vi "Check VISA instrument.vi"(8 "error in (no error)":errorcluster, 10 "visa instrumnet string":string) -> (0 "error out":errorcluster, 3 "error":bool caption="error indicator")   [LabVIEW 2021]
uses:
  <vilib>/regexp/Match Regular Expression.xnode
panel:
  out "device response":string
  out "Read ∆ Time (ms)":dbl format="%.4f"
  out "identifier string":string
  out "VISA instruments":refnum<visa-resource-name>
  in  "included VISA instruments":string[](array[string])=["gpib", "asrl", "com", "end of list"]
  # "end of list should be the last item"
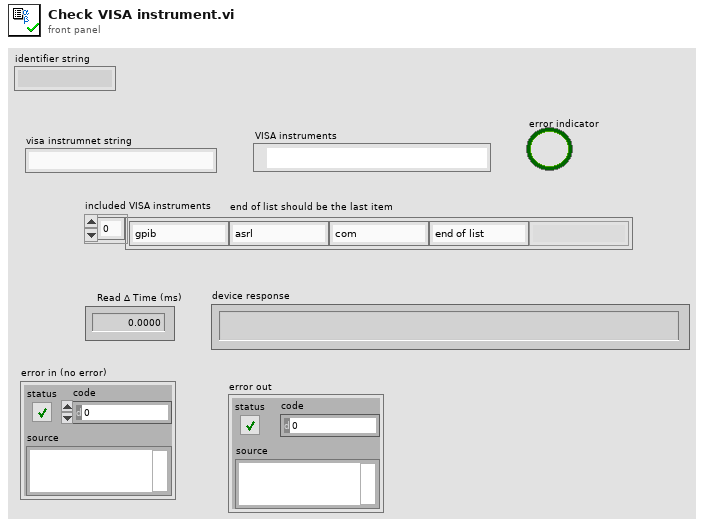
[diagram p1: front panel]
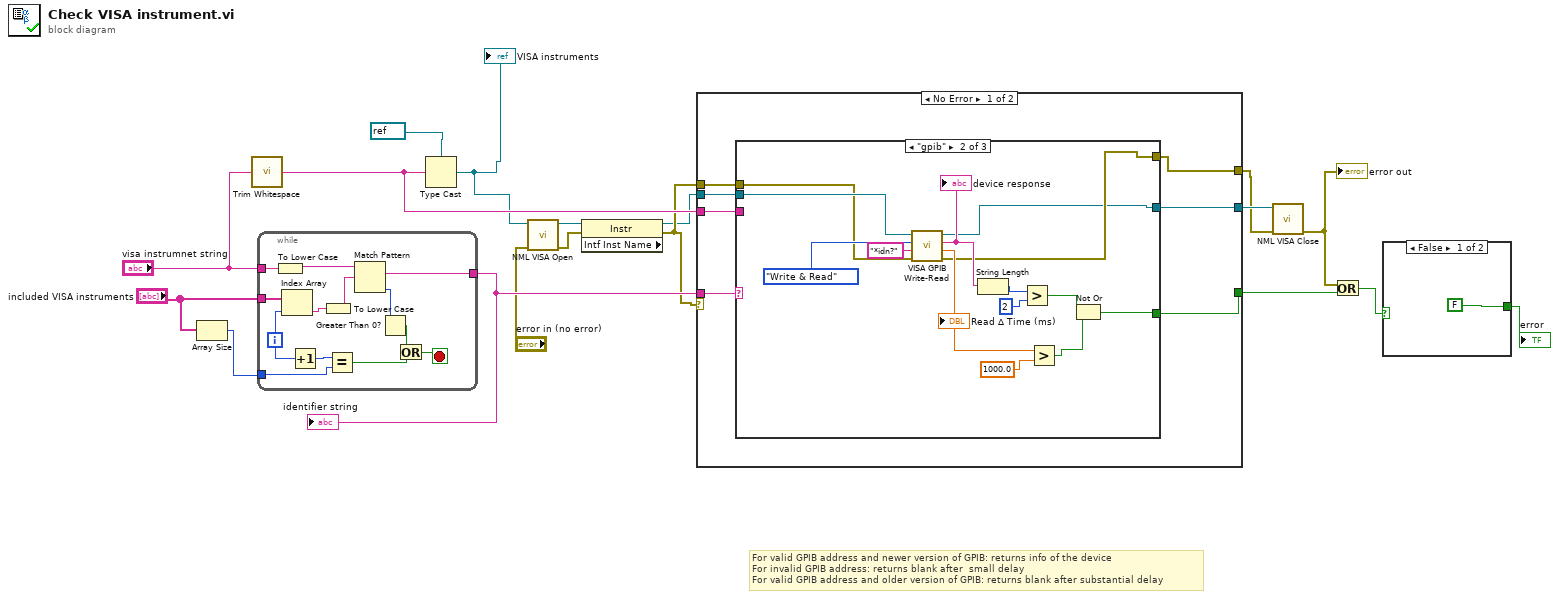
[diagram p0: block diagram]
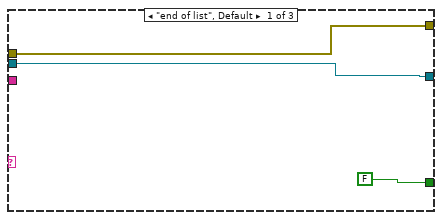
[diagram p2: hidden frame]
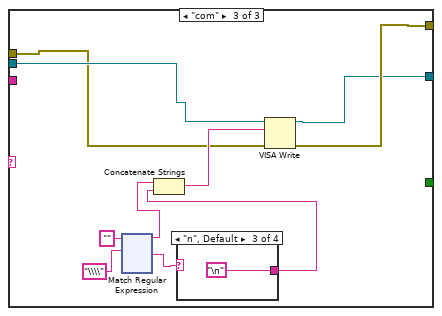
[diagram p3: hidden frame]
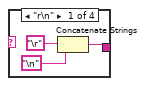
[diagram p4: hidden frame]
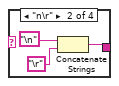
[diagram p5: hidden frame]
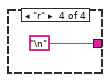
[diagram p6: hidden frame]
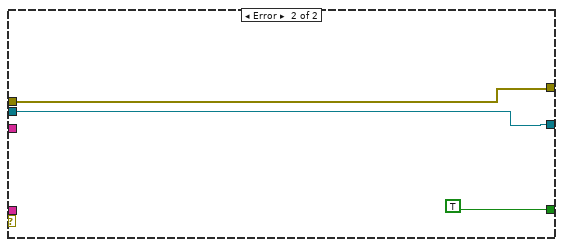
[diagram p7: hidden frame]
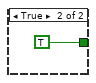
[diagram p8: hidden frame]
diagram:
  # "For valid GPIB address and newer version of GPIB: returns info of the device\nFor invalid GPIB address: returns blank after  small delay\nFor valid GPIB address and older version of GPIB: returns blank after substantial delay"
  n1 = Array Size(array="included VISA instruments") -> (size(s)=w17:i32)
  n2 = call <vilib>:"Trim Whitespace.vi"("string"="visa instrumnet string") -> ("trimmed string"=w13:string)  [unwired: 1 in]
  n3 = while {
    tunnel: "visa instrumnet string" -> [w31]
    tunnel: "included VISA instruments" -> [w30]
    tunnel: [w25] -> w12
    tunnel: w17 -> [w20]
    i -> [w22]
    stop <- w23 stop-if-true
    n4 = To Lower Case(string=w31) -> (all lower case string=w27:string)
    n5 = Index Array(array=w30, index=w22) -> (element=w29:string)
    n6 = Increment(x=w22) -> (x+1=w21:i32)
    n7 = To Lower Case(string=w29) -> (all lower case string=w28:string)
    n8 = Equal?(x=w21, y=w20) -> (x = y?=w19:bool)
    n9 = Match Pattern(string=w27, regular expression=w28) -> (match substring=w25:string, offset past match=w26:i32)  [unwired: 1 in, 2 out]
    n10 = Greater Than 0?(x=w26) -> (x > 0?=w24:bool)
    n11 = Or(x=w24, y=w19) -> (x .or. y?=w23:bool)
  }
  "identifier string" <- w12
  n12 = Type Cast(type=refnum<visa-resource-name> refnum ("VISA resource name"), x=w13) -> (*(type *) &x=w11:refnum<visa-resource-name>)
  "VISA instruments" <- w11
  n13 = call "NML VISA Open.vi"("error in (no error)"="error in (no error)", "VISA resource name"=w11) -> ("error out"=w8:errorcluster, "VISA resource name out"=w10:refnum<visa-resource-name>)  [unwired: 8 in]
  n14 = property class="Instr" props=["Intf Inst Name"](reference=w10, error in=w8) -> (reference out=w6:refnum<visa-resource-name>, error out=w7:errorcluster)  [unwired: 1 out]
  n15 = case shown="No Error" w7 {
    tunnel: w7 -> [w38 w193]
    tunnel: w13 -> [w37 _]
    tunnel: [w36 w193] -> w2
    tunnel: w12 -> [w35 _]
    tunnel: w6 -> [w34 w191]
    tunnel: [w33 TRUE] -> w5
    tunnel: [w32 w191] -> w3
    frame No Error {
      n16 = case shown="\"gpib\"" w35 {
        tunnel: [w41 w46 w65] -> w36
        tunnel: w34 -> [w39 w48 w64]
        tunnel: w38 -> [w41 w47 w58]
        tunnel: w37 -> [_ _ _]
        tunnel: [FALSE w42 _] -> w33
        tunnel: [w39 w45 w56] -> w32
        frame "end of list", Default {
        }
        frame "gpib" {
          n17 = call "VISA GPIB Write-Read.vi"("error in (no error)"=w47, "Command"="*idn?", "Action"=enum16{"Write", "Read", "Write & Read"}."Write & Read", "VISA resource name"=w48) -> ("error out"=w46:errorcluster, "Read ∆ Time [ms]"=w50:dbl, "String Returned"=w53:string, "dup VISA Session"=w45:refnum<visa-resource-name>)  [unwired: 4 in]
          "Read ∆ Time (ms)" <- w50
          "device response" <- w53
          n18 = String Length(string=w53) -> (length=w52:i32)
          n19 = Greater?(x=w52, y=2) -> (0:w44:bool)
          n20 = Greater?(x=w50, y=1000.0) -> (0:w43:bool)
          n21 = Not Or(1:w43, 2:w44) -> (0:w42:bool)
        }
        frame "com" {
          n22 = xnode "Match Regular Expression"("input string"="", "regular expression"="\\\\") -> ("before match"=w60:string, "after match"=w61:string)  [unwired: 4 in, 3 out]
          n23 = case shown="\"n\", Default" w61 {
            tunnel: [w66 w71 "\n" "\n"] -> w59
            frame "r\n" {
              n24 = Concatenate Strings("\r", "\n") -> (w66:string)
            }
            frame "n\r" {
              n25 = Concatenate Strings("\n", "\r") -> (w71:string)
            }
            frame "n", Default {
            }
            frame "r" {
            }
          }
          n26 = Concatenate Strings(w60, w59) -> (w63:string)
          n27 = VISA Write(VISA resource name=w64, write buffer=w63, error in (no error)=w58) -> (VISA resource name out=w56:refnum<visa-resource-name>, error out=w65:errorcluster)  [unwired: 1 out]
        }
      }
    }
    frame Error {
    }
  }
  n28 = call "NML VISA Close.vi"("Error In"=w2, "VISA resource name"=w3) -> ("Error Out"=w1:errorcluster)  [unwired: 9 in]
  "error out" <- w1
  n29 = Or(x=w1, y=w5) -> (x .or. y?=w4:bool)
  n30 = case shown="False" w4 {
    tunnel: [FALSE ("error") TRUE ("error")] -> w14
    frame False {
    }
    frame True {
    }
  }
  "error" <- w14
